vi "Host_SurfaceAutoApproach.vi"() -> ()   [LabVIEW 2014]
uses:
  <vilib>/Instr/_visa.llb/VISA Configure Serial Port (Instr).vi
  <vilib>/FPGAPlugInAG/PCIe-7851R/niLvFpga_Open_PCIe-7851R.vi
  <vilib>/rvi/interface/common/dynamic/niFpgaDynamicAddResources.vi
  <vilib>/Utility/error.llb/Error Cluster From Error Code.vi
  <vilib>/rvi/errors/niLvFpgaAdjustHostInterfaceError.vi
  <vilib>/FPGAPlugInAG/Dynamic/niLvFpga_Close_Dynamic.vi
  <vilib>/rvi/interface/nirviOpenFPGA/nirviOpenFPGA.xnode
  FPGA Bitfiles/MetalGrowthv1_FPGATarget_FPGASingleApproa_auVMqFU+myY.lvbitx
  <vilib>/rvi/interface/nirviReadWriteControl/nirviReadWriteControl.xnode
  <vilib>/rvi/interface/nirviCloseFPGA/nirviCloseFPGA.xnode
  NiFpgaLv.dll
  <vilib>/rvi/interface/Simulation/niFpgaSimulationCallBeginRW.vi
panel:
  in  "ThresMultiplier":i32
  in  "Sleep us":i32
  out "PIZPosDia":i16(graph)
  out "CurrDia":i16(graph)
  out "Curr":i16
  out "ZRealPos":i16
  out "ZCalPos":i32
  in  "stop":bool
  out "RoughZPos?":dbl
  in  "UseMemoryPos?":bool=TRUE
  in  "ContinuousReapproach":bool
  in  "RoughZInitPos":dbl format="%#_13g"
  in  "RoughZ":refnum<visa-resource-name>
  out "Error?":string
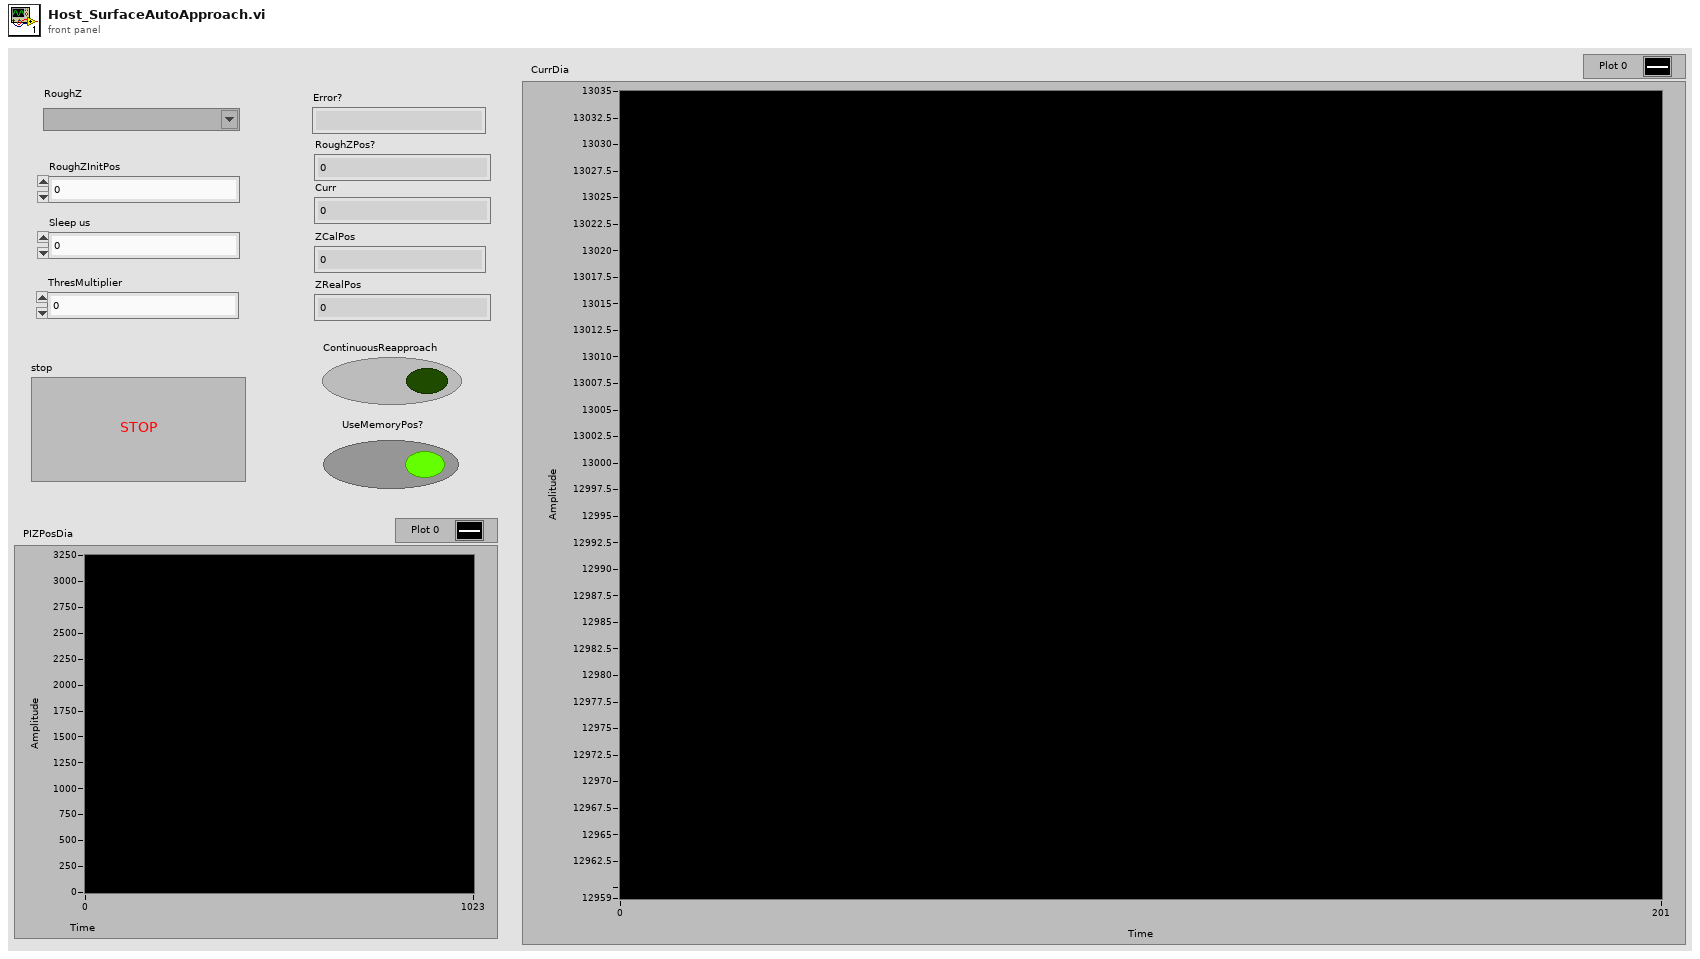
[diagram p1: front panel]
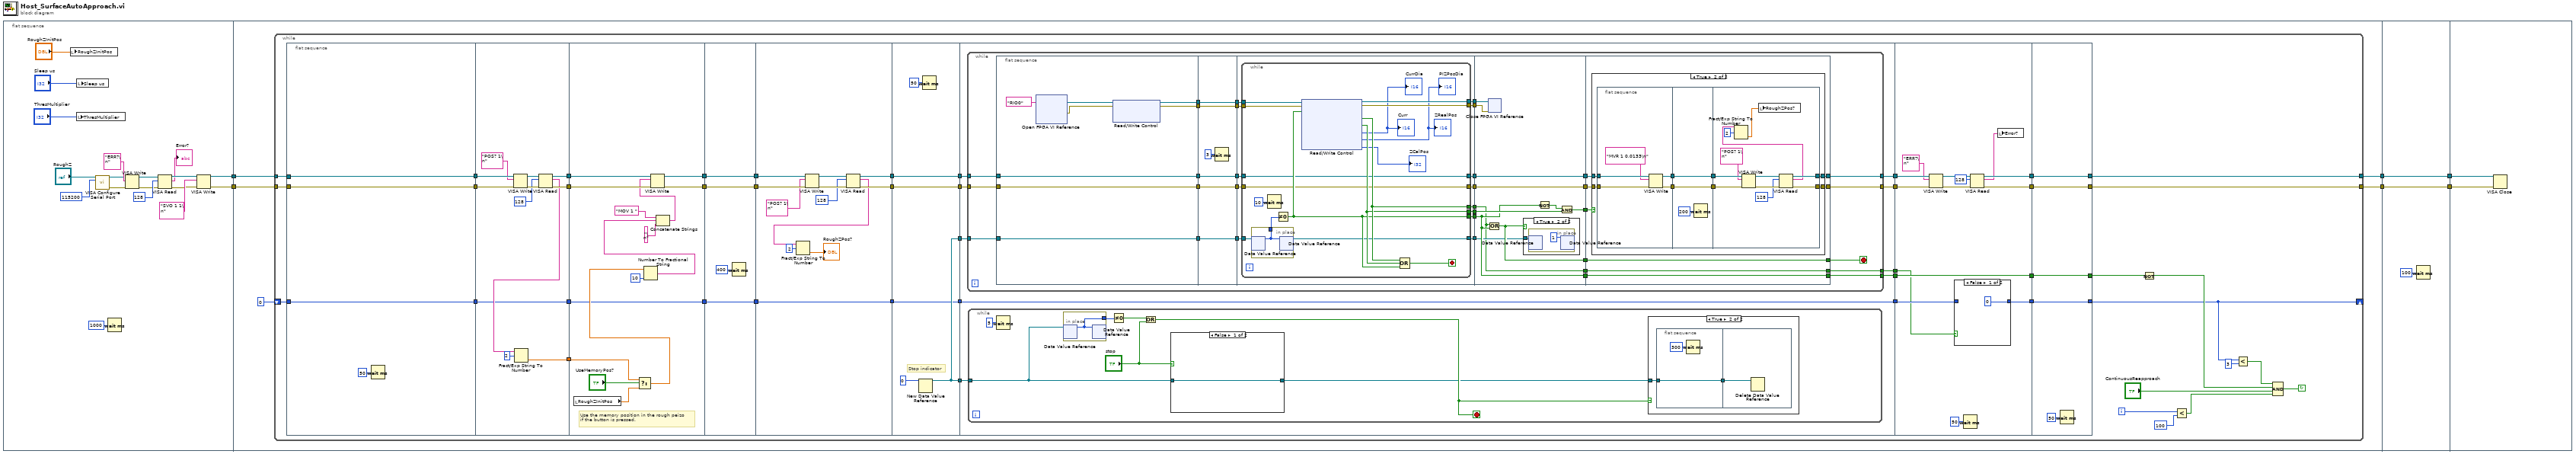
[diagram p0: block diagram]
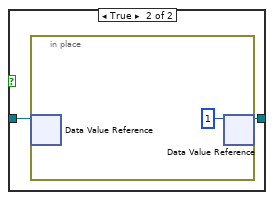
[diagram p3: hidden frame]
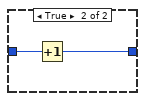
[diagram p6: hidden frame]
diagram:
  n1 = flat-sequence {
    tunnel: [w10] -> w6
    tunnel: [w9] -> w5
    tunnel: [w28] -> w4
    tunnel: [w27] -> w3
    tunnel: w6 -> [w26]
    tunnel: w5 -> [w25]
    tunnel: [w304] -> w2
    tunnel: w4 -> [w304]
    tunnel: [w303] -> w1
    tunnel: w3 -> [w303]
    tunnel: w2 -> [w306]
    tunnel: w1 -> [w305]
    frame #0 {
      n2 = local write "RoughZInitPos"("RoughZInitPos") -> ()
      n3 = local write "ThresMultiplier"("ThresMultiplier") -> ()
      n4 = local write "Sleep us"("Sleep us") -> ()
      n5 = call-poly "VISA Configure Serial Port"("VISA resource name"="RoughZ", "baud rate (9600)"=u32 115200) -> ("VISA resource name out"=w13:refnum<visa-resource-name>, "error out"=w14:errorcluster)  [unwired: 12 in]
      n6 = Wait (ms)(milliseconds to wait=u32 1000) -> ()  [unwired: 1 out]
      n7 = VISA Write(VISA resource name=w13, write buffer="ERR?\n", error in (no error)=w14) -> (VISA resource name out=w16:refnum<visa-resource-name>, error out=w17:errorcluster)  [unwired: 1 out]
      n8 = VISA Read(VISA resource name=w16, byte count=u32 128, error in (no error)=w17) -> (VISA resource name out=w20:refnum<visa-resource-name>, read buffer=→"Error?":string, error out=w21:errorcluster)  [unwired: 1 out]
      n9 = VISA Write(VISA resource name=w20, write buffer="SVO 1 1\n", error in (no error)=w21) -> (VISA resource name out=w10:refnum<visa-resource-name>, error out=w9:errorcluster)  [unwired: 1 out]
    }
    frame #1 {
      n10 = while {
        shift-right: [w36] -> _
        shift-left: 0 -> [w46]
        tunnel: [w34] -> w28
        tunnel: [w33] -> w27
        tunnel: w26 -> [w32]
        tunnel: w25 -> [w31]
        i -> [w55]
        stop <- w49 continue-if-true
        n11 = flat-sequence {
          tunnel: [w76] -> w74
          tunnel: [w75] -> w73
          tunnel: w46 -> [w78]
          tunnel: [w78] -> w45
          tunnel: w32 -> [w76]
          tunnel: w31 -> [w75]
          tunnel: w74 -> [w90]
          tunnel: [w86] -> w72
          tunnel: w73 -> [w89]
          tunnel: [w85] -> w71
          tunnel: [w80] -> w70
          tunnel: w45 -> [w79]
          tunnel: [w79] -> w44
          tunnel: w72 -> [w104]
          tunnel: w71 -> [w103]
          tunnel: [w97] -> w69
          tunnel: [w96] -> w68
          tunnel: w70 -> [w94]
          tunnel: w44 -> [w91]
          tunnel: [w91] -> w41
          tunnel: w69 -> [w108]
          tunnel: w68 -> [w107]
          tunnel: [w108] -> w67
          tunnel: [w107] -> w66
          tunnel: [w105] -> w42
          tunnel: w41 -> [w105]
          tunnel: w67 -> [w120]
          tunnel: w66 -> [w119]
          tunnel: [w114] -> w65
          tunnel: [w113] -> w64
          tunnel: [w109] -> w43
          tunnel: w42 -> [w109]
          tunnel: [w126] -> w63
          tunnel: [w125] -> w62
          tunnel: [w122] -> w61
          tunnel: [w122] -> w60
          tunnel: w64 -> [w125]
          tunnel: w65 -> [w126]
          tunnel: w43 -> [w121]
          tunnel: [w121] -> w40
          tunnel: w63 -> [w135]
          tunnel: w62 -> [w134]
          tunnel: w61 -> [w133]
          tunnel: w60 -> [w132]
          tunnel: [w131] -> w59
          tunnel: [w130] -> w58
          tunnel: [w129] -> w53
          tunnel: w40 -> [w128]
          tunnel: [w128] -> w39
          tunnel: [w127] -> w38
          tunnel: w59 -> [w293]
          tunnel: w58 -> [w292]
          tunnel: [w287] -> w57
          tunnel: [w286] -> w56
          tunnel: w53 -> [w282]
          tunnel: [w282] -> w52
          tunnel: w39 -> [w283]
          tunnel: w38 -> [w280]
          tunnel: [w281] -> w37
          tunnel: [w300] -> w48
          tunnel: [w299] -> w34
          tunnel: [w298] -> w33
          tunnel: w52 -> [w300]
          tunnel: w56 -> [w298]
          tunnel: w57 -> [w299]
          tunnel: w37 -> [w297]
          tunnel: [w297] -> w36
          frame #0 {
            n12 = Wait (ms)(milliseconds to wait=u32 50) -> ()  [unwired: 1 out]
          }
          frame #1 {
            n13 = VISA Write(VISA resource name=w90, write buffer="POS? 1\n", error in (no error)=w89) -> (VISA resource name out=w88:refnum<visa-resource-name>, error out=w87:errorcluster)  [unwired: 1 out]
            n14 = VISA Read(VISA resource name=w88, byte count=u32 128, error in (no error)=w87) -> (VISA resource name out=w86:refnum<visa-resource-name>, read buffer=w82:string, error out=w85:errorcluster)  [unwired: 1 out]
            n15 = Fract/Exp String To Number(string=w82, offset=2) -> (number=w80:dbl)  [unwired: 2 in, 1 out]
          }
          frame #2 {
            # "Use the memory position in the rough peizo\nif the button is pressed."
            n16 = local read "RoughZInitPos"() -> (w93:dbl)
            n17 = Select(t=w94, s="UseMemoryPos?", f=w93) -> (s? t:f=w92:dbl)
            n18 = Number To Fractional String(number=w92, precision (6)=i16 10) -> (F-format string=w100:string)  [unwired: 2 in]
            n19 = Concatenate Strings("MOV 1 " ("string"), w100, "\n" ("string")) -> (w102:string)
            n20 = VISA Write(VISA resource name=w104, write buffer=w102, error in (no error)=w103) -> (VISA resource name out=w97:refnum<visa-resource-name>, error out=w96:errorcluster)  [unwired: 1 out]
          }
          frame #3 {
            n21 = Wait (ms)(milliseconds to wait=u32 400) -> ()  [unwired: 1 out]
          }
          frame #4 {
            n22 = VISA Write(VISA resource name=w120, write buffer="POS? 1\n", error in (no error)=w119) -> (VISA resource name out=w117:refnum<visa-resource-name>, error out=w116:errorcluster)  [unwired: 1 out]
            n23 = VISA Read(VISA resource name=w117, byte count=u32 128, error in (no error)=w116) -> (VISA resource name out=w114:refnum<visa-resource-name>, read buffer=w112:string, error out=w113:errorcluster)  [unwired: 1 out]
            n24 = Fract/Exp String To Number(string=w112, offset=2) -> (number=→"RoughZPos?":dbl)  [unwired: 2 in, 1 out]
          }
          frame #5 {
            # "Stop indicator"
            n25 = New Data Value Reference(data value=0) -> (data value reference=w122:refnum<data-value>)  [unwired: 1 in, 1 out]
            n26 = Wait (ms)(milliseconds to wait=u32 50) -> ()  [unwired: 1 out]
          }
          frame #6 {
            n27 = while {
              tunnel: w135 -> [w184]
              tunnel: w134 -> [w183]
              tunnel: w132 -> [w182]
              tunnel: [w168] -> w131
              tunnel: [w167] -> w130
              tunnel: [w165] -> w129
              tunnel: [w153] -> w127
              stop <- w169 stop-if-true
              n28 = flat-sequence {
                tunnel: w184 -> [w191]
                tunnel: w183 -> [w190]
                tunnel: [w186] -> w164
                tunnel: [w185] -> w162
                tunnel: [w192] -> w160
                tunnel: w182 -> [w192]
                tunnel: [w191] -> w158
                tunnel: [w190] -> w156
                tunnel: w164 -> [w198]
                tunnel: [w198] -> w163
                tunnel: w162 -> [w197]
                tunnel: [w197] -> w161
                tunnel: w160 -> [w196]
                tunnel: [w196] -> w159
                tunnel: w158 -> [w195]
                tunnel: [w195] -> w157
                tunnel: w156 -> [w194]
                tunnel: [w194] -> w155
                tunnel: w163 -> [w211]
                tunnel: w161 -> [w210]
                tunnel: w159 -> [w209]
                tunnel: w157 -> [w208]
                tunnel: w155 -> [w207]
                tunnel: [w206] -> w181
                tunnel: [w205] -> w180
                tunnel: [w204] -> w179
                tunnel: [w203] -> w178
                tunnel: [w202] -> w177
                tunnel: [w201] -> w176
                tunnel: [w200] -> w175
                tunnel: [w199] -> w174
                tunnel: w181 -> [w230]
                tunnel: w180 -> [w237]
                tunnel: w179 -> [w232]
                tunnel: w178 -> [w240]
                tunnel: w177 -> [w239]
                tunnel: w176 -> [w234]
                tunnel: w175 -> [w235]
                tunnel: w174 -> [w231]
                tunnel: [w236] -> w173
                tunnel: [w235] -> w172
                tunnel: [w234] -> w171
                tunnel: [w233] -> w170
                tunnel: [w232] -> w166
                tunnel: [w230] -> w154
                tunnel: w173 -> [w250]
                tunnel: w172 -> [w249]
                tunnel: w171 -> [w248]
                tunnel: w170 -> [w247]
                tunnel: [w247] -> w169
                tunnel: [w246] -> w168
                tunnel: [w245] -> w167
                tunnel: w166 -> [w244]
                tunnel: [w244] -> w165
                tunnel: w154 -> [w243]
                tunnel: [w243] -> w153
                frame #0 {
                  n29 = xnode "Open FPGA VI Reference"("resource name"=tag "RIO0") -> ("FPGA VI Reference Out"=w188:refnum<k20>, "error out"=w187:errorcluster)  [unwired: 1 in]
                  n30 = xnode "Read/Write Control"("FPGA VI Reference In"=w188, "error in"=w187) -> ("FPGA VI Reference Out"=w186:refnum<k20>, "error out"=w185:errorcluster)  [unwired: 2 in]
                }
                frame #1 {
                  n31 = Wait (ms)(milliseconds to wait=u32 3) -> ()  [unwired: 1 out]
                }
                frame #2 {
                  n32 = while {
                    tunnel: w211 -> [w228]
                    tunnel: w210 -> [w227]
                    tunnel: w209 -> [w226]
                    tunnel: w208 -> [w218]
                    tunnel: w207 -> [w217]
                    tunnel: [w223] -> w206
                    tunnel: [w222] -> w205
                    tunnel: [w221] -> w204
                    tunnel: [w220] -> w203
                    tunnel: [w219] -> w202
                    tunnel: [w218] -> w200
                    tunnel: [w217] -> w201
                    tunnel: [w216] -> w199
                    stop <- w224 stop-if-true
                    n33 = in-place {
                      in-place-border: [w229] -> w225
                      n34 = in-place-dvr #1(w226) -> (w229:i32)  [unwired: 1 out]
                      n35 = in-place-dvr #1(w229) -> (w216:refnum<data-value>)  [unwired: 1 out]
                    }
                    n36 = Wait (ms)(milliseconds to wait=u32 10) -> ()  [unwired: 1 out]
                    n37 = Not Equal To 0?(x=w225) -> (x != 0?=w221:bool)
                    n38 = xnode "Read/Write Control"("FPGA VI Reference In"=w228, "error in"=w227, "stop"=w221) -> ("FPGA VI Reference Out"=w220:refnum<k20>, "error out"=w219:errorcluster, "Approached?"=w223:bool, "PIZRangeExceeded?"=w222:bool, "PresCurr"=→"CurrDia" →"Curr":i16, "RealPIZPos"=→"PIZPosDia" →"ZRealPos":i16, "ZCalPos"=→"ZCalPos":i32)
                    n39 = Compound Arithmetic op=OR(w223, w222, w221) -> (w224:bool)
                  }
                }
                frame #3 {
                  n40 = Or(x=w230, y=w232) -> (x .or. y?=w233:bool)
                  n41 = xnode "Close FPGA VI Reference"("FPGA VI Reference In"=w240, "error in"=w239) -> ()  [unwired: 1 out]
                  n42 = case shown="True" w233 {
                    tunnel: w231 -> [_ w241]
                    frame False {
                    }
                    frame True {
                      n43 = in-place {
                        n44 = in-place-dvr #2(w241) -> ()  [unwired: 2 out]
                        n45 = in-place-dvr #2(1 ("data value")) -> ()  [unwired: 2 out]
                      }
                    }
                  }
                  n46 = Not(x=w232) -> (.not. x?=w238:bool)
                  n47 = And(x=w238, y=w237) -> (x .and. y?=w236:bool)
                }
                frame #4 {
                  n48 = case shown="True" w250 {
                    tunnel: w249 -> [w252 w260]
                    tunnel: w248 -> [w251 w259]
                    tunnel: [w252 w254] -> w246
                    tunnel: [w251 w253] -> w245
                    frame False {
                    }
                    frame True {
                      n49 = flat-sequence {
                        tunnel: w260 -> [w265]
                        tunnel: w259 -> [w264]
                        tunnel: [w262] -> w258
                        tunnel: [w261] -> w257
                        tunnel: w258 -> [w268]
                        tunnel: w257 -> [w267]
                        tunnel: [w268] -> w256
                        tunnel: [w267] -> w255
                        tunnel: w256 -> [w279]
                        tunnel: w255 -> [w278]
                        tunnel: [w273] -> w254
                        tunnel: [w272] -> w253
                        frame #0 {
                          n50 = VISA Write(VISA resource name=w265, write buffer="MVR 1 0.0133\n", error in (no error)=w264) -> (VISA resource name out=w262:refnum<visa-resource-name>, error out=w261:errorcluster)  [unwired: 1 out]
                        }
                        frame #1 {
                          n51 = Wait (ms)(milliseconds to wait=u32 200) -> ()  [unwired: 1 out]
                        }
                        frame #2 {
                          n52 = VISA Write(VISA resource name=w279, write buffer="POS? 1\n", error in (no error)=w278) -> (VISA resource name out=w276:refnum<visa-resource-name>, error out=w275:errorcluster)  [unwired: 1 out]
                          n53 = VISA Read(VISA resource name=w276, byte count=u32 128, error in (no error)=w275) -> (VISA resource name out=w273:refnum<visa-resource-name>, read buffer=w271:string, error out=w272:errorcluster)  [unwired: 1 out]
                          n54 = Fract/Exp String To Number(string=w271, offset=2) -> (number=w269:dbl)  [unwired: 2 in, 1 out]
                          n55 = local write "RoughZPos?"(w269) -> ()
                        }
                      }
                    }
                  }
                }
              }
            }
            n56 = while {
              tunnel: w133 -> [w141]
              stop <- w137 stop-if-true
              n57 = Wait (ms)(milliseconds to wait=u32 5) -> ()  [unwired: 1 out]
              n58 = in-place {
                in-place-border: [w148] -> w140
                n59 = in-place-dvr #3(w141) -> (w148:i32)  [unwired: 1 out]
                n60 = in-place-dvr #3(w148) -> ()  [unwired: 2 out]
              }
              n61 = Not Equal To 0?(x=w140) -> (x != 0?=w139:bool)
              n62 = Or(x=w139, y="stop") -> (x .or. y?=w137:bool)
              n63 = case shown="False" "stop" {
                tunnel: w141 -> [w149 w151]
                tunnel: [w149 w150] -> w136
                frame False {
                }
                frame True {
                  n64 = in-place {
                    n65 = in-place-dvr #4(w151) -> ()  [unwired: 2 out]
                    n66 = in-place-dvr #4(1 ("data value")) -> (w150:refnum<data-value>)  [unwired: 1 out]
                  }
                }
              }
              n67 = case shown="True" w137 {
                tunnel: w136 -> [_ w144]
                frame False {
                }
                frame True {
                  n68 = flat-sequence {
                    tunnel: w144 -> [w145]
                    tunnel: [w145] -> w143
                    tunnel: w143 -> [w147]
                    frame #0 {
                      n69 = Wait (ms)(milliseconds to wait=u32 300) -> ()  [unwired: 1 out]
                    }
                    frame #1 {
                      n70 = Delete Data Value Reference(data value reference=w147) -> ()  [unwired: 1 in, 2 out]
                    }
                  }
                }
              }
            }
          }
          frame #7 {
            n71 = VISA Write(VISA resource name=w293, write buffer="ERR?\n", error in (no error)=w292) -> (VISA resource name out=w291:refnum<visa-resource-name>, error out=w290:errorcluster)  [unwired: 1 out]
            n72 = case shown="False" w280 {
              tunnel: w283 -> [_ w296]
              tunnel: [0 w295] -> w281
              frame False {
              }
              frame True {
                n73 = Increment(x=w296) -> (x+1=w295:i32)
              }
            }
            n74 = Wait (ms)(milliseconds to wait=u32 50) -> ()  [unwired: 1 out]
            n75 = VISA Read(VISA resource name=w291, byte count=u32 128, error in (no error)=w290) -> (VISA resource name out=w287:refnum<visa-resource-name>, read buffer=w285:string, error out=w286:errorcluster)  [unwired: 1 out]
            n76 = local write "Error?"(w285) -> ()
          }
          frame #8 {
            n77 = Wait (ms)(milliseconds to wait=u32 50) -> ()  [unwired: 1 out]
          }
        }
        n78 = Not(x=w48) -> (.not. x?=w47:bool)
        n79 = Less?(x=w55, y=100) -> (x < y?=w50:bool)
        n80 = Less?(x=w36, y=3) -> (x < y?=w30:bool)
        n81 = Compound Arithmetic op=AND(w30, w47, "ContinuousReapproach", w50) -> (w49:bool)
      }
    }
    frame #2 {
      n82 = Wait (ms)(milliseconds to wait=u32 100) -> ()  [unwired: 1 out]
    }
    frame #3 {
      n83 = VISA Close(VISA resource name=w306, error in (no error)=w305) -> ()  [unwired: 1 out]
    }
  }
